vi "Calculate Code Sweep Transition Settings.vi"(9 "Code transition type":T1 items=["Negative", "Bipolar zero", "Positive"], 10 "Sweep transition settings":T3) -> (0 "Sweep configurations":T2, 1 "Ideal LSB":dbl, 2 "Ideal transition":dbl, 3 "Code before transition":u32)   [LabVIEW 2021, in "Full Scale Error_ADC.lvlib"]
uses:
  Full Scale Error_ADC.lvlib
  Controls/Sweep Transition Settings.ctl
  Controls/Sweep Configurations.ctl
  Controls/Code Transition Type.ctl
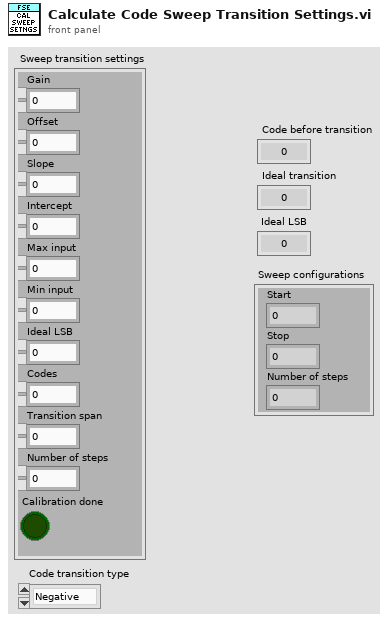
[diagram p1: front panel]
types:
  T1 = typedef "Full Scale Error_ADC.lvlib/Code Transition Type.ctl" = u16
  T2 = typedef "Full Scale Error_ADC.lvlib/Sweep Configurations.ctl" = cluster{"Start":dbl, "Stop":dbl, "Number of steps":i32}
  T3 = typedef "Full Scale Error_ADC.lvlib/Sweep Transition Settings.ctl" = cluster{"Gain":dbl, "Offset":dbl, "Slope":dbl, "Intercept":dbl, "Max input":dbl, "Min input":dbl, "Ideal LSB":dbl, "Codes":dbl, "Transition span ":dbl, "Number of steps":i32, "Calibration done":bool}
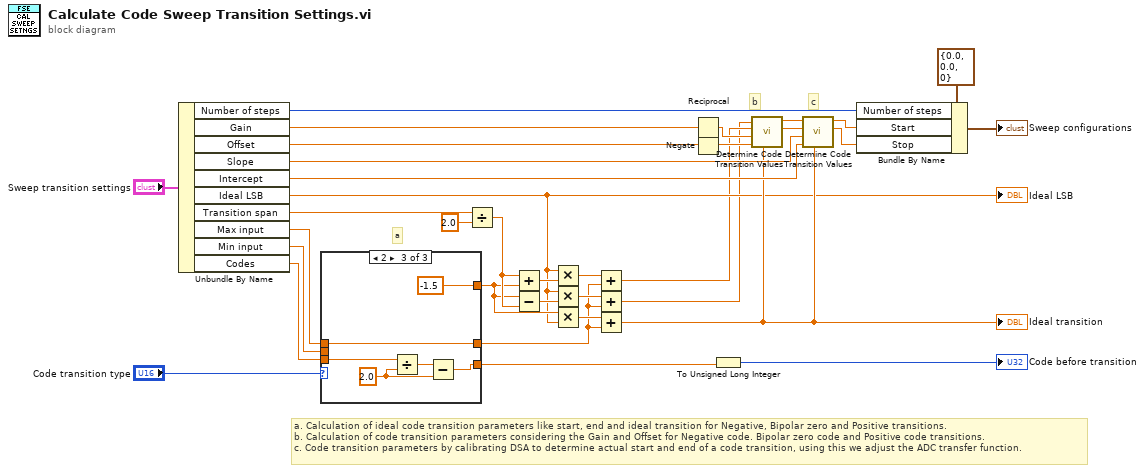
[diagram p0: block diagram]
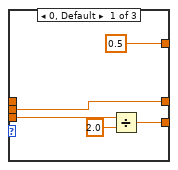
[diagram p2: hidden frame]
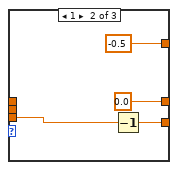
[diagram p3: hidden frame]
diagram:
  # "a. Calculation of ideal code transition parameters like start, end and ideal transition for Negative, Bipolar zero and Positive transitions.\nb. Calculation of code transition parameters considering the Gain and Offset for Negative code. Bipolar zero code and Positive code transitions.\nc. Code transition parameters by calibrating DSA to determine actual start and end of a code transition, using this we adjust the ADC transfer function."
  # "c"
  # "b"
  # "a"
  n1 = Unbundle By Name("Sweep transition settings") -> ("Number of steps"=w20:i32, "Gain"=w33:dbl, "Offset"=w32:dbl, "Slope"=w27:dbl, "Intercept"=w26:dbl, "Ideal LSB"=w3:dbl, "Transition span"=w7:dbl, "Max input"=w4:dbl, "Min input"=w5:dbl, "Codes"=w6:dbl)
  "Ideal LSB" <- w3
  n2 = case shown="2" "Code transition type" {
    tunnel: [0.5 -0.5 -1.5] -> w14
    tunnel: [w38 0.0 ("Max Input") w48] -> w10
    tunnel: w5 -> [w38 _ _]
    tunnel: w4 -> [_ _ w48]
    tunnel: w6 -> [w37 w41 w47]
    tunnel: [w35 w40 w44] -> w8
    frame 0, Default {
      n3 = Divide(x=w37, y=2.0) -> (x/y=w35:dbl)
    }
    frame 1 {
      n4 = Decrement(x=w41) -> (x-1=w40:dbl)
    }
    frame 2 {
      w45 = 2.0 ("y")
      n5 = Divide(x=w47, y=w45) -> (x/y=w46:dbl)
      n6 = Subtract(x=w46, y=w45) -> (x-y=w44:dbl)
    }
  }
  n7 = Divide(x=w7, y=2.0) -> (x/y=w17:dbl)
  n8 = Add(x=w17, y=w14) -> (x+y=w16:dbl)
  n9 = Subtract(x=w14, y=w17) -> (x-y=w15:dbl)
  n10 = Multiply(x=w3, y=w16) -> (x*y=w13:dbl)
  n11 = Multiply(x=w3, y=w15) -> (x*y=w12:dbl)
  n12 = Multiply(x=w14, y=w3) -> (x*y=w11:dbl)
  n13 = Add(x=w13, y=w10) -> (x+y=w2:dbl)
  n14 = Add(x=w12, y=w10) -> (x+y=w1:dbl)
  n15 = Add(x=w11, y=w10) -> (x+y=w9:dbl)
  "Ideal transition" <- w9
  n16 = Reciprocal(x=w33) -> (1/x=w31:dbl)
  n17 = Negate(x=w32) -> (-x=w30:dbl)
  n18 = To Unsigned Long Integer(number=w8) -> (unsigned 32bit integer=→"Code before transition":u32)
  n19 = call "Determine Code Transition Values.vi"("Transition"=w9, "Intercept"=w30, "Slope"=w31, "End"=w2, "Start"=w1) -> ("Actual end"=w28:dbl, "Actual start"=w29:dbl)  [unwired: 4 in, 1 out]
  n20 = call "Determine Code Transition Values.vi"("Transition"=w9, "Intercept"=w26, "Slope"=w27, "End"=w28, "Start"=w29) -> ("Actual end"=w22:dbl, "Actual start"=w23:dbl)  [unwired: 4 in, 1 out]
  n21 = Bundle By Name(cluster=T2 {"Start"=0.0, "Stop"=0.0, "Number of steps"=0} ("Sweep Configurations"), "Number of steps"=w20, "Start"=w23, "Stop"=w22) -> (→"Sweep configurations":T2)
